vi "Register for Triggered Log State Change Event.vi"(8 "error in (no error)":errorcluster, 9 "User Data":variant, 10 "State Change Callback":refnum<vi>, 11 "Triggered Log in":refnum<class "Triggered Log.lvclass">) -> (0 "error out":errorcluster, 3 "Triggered Log out":refnum<class "Triggered Log.lvclass">)   [LabVIEW 2012, in "Triggered Log.lvclass"]
uses:
  Triggered Log.lvclass
  Triggered Log.lvclass/Triggered Log.ctl
  Triggered Log State Change Event Registration.ctl
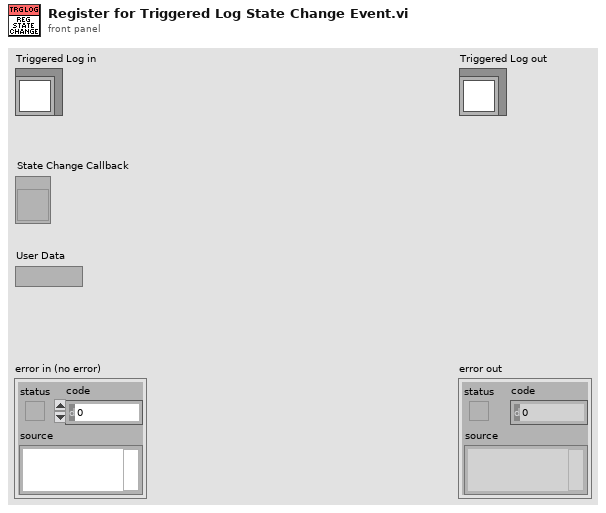
[diagram p1: front panel]
types:
  T1 = typedef "Triggered Log.lvclass/Triggered Log State Change Event Registration.ctl" = cluster{"Callback":refnum<vi>, "User Data":variant}
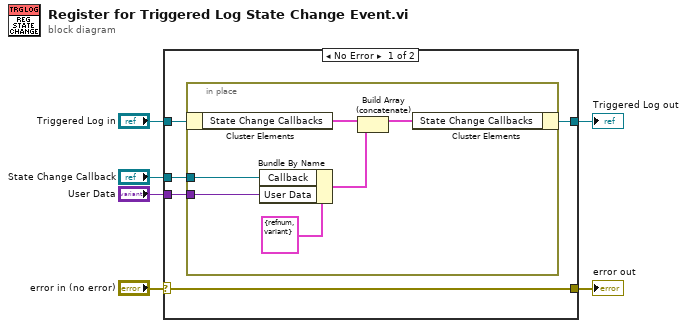
[diagram p0: block diagram]
diagram:
  n1 = case shown="No Error" "error in (no error)" {
    selector: "error in (no error)" -> [w9 w19]
    tunnel: [w9 w19] -> w5
    tunnel: [w10 w18] -> w3
    tunnel: "Triggered Log in" -> [w11 w18]
    tunnel: "State Change Callback" -> [w8 _]
    tunnel: "User Data" -> [w7 _]
    frame No Error {
      n2 = in-place {
        in-place-border: w8 -> [w14]
        in-place-border: w7 -> [w13]
        n3 = in-place-cluster #1(w11) -> ("State Change Callbacks"=w17:T1[])
        n4 = Bundle By Name(cluster=T1 {"Callback"=refnum, "User Data"=variant} ("Trigger Event Registration"), "Callback"=w14, "User Data"=w13) -> (w12:T1)
        n5 = Build Array (concatenate)(w17, w12) -> (w16:T1[])
        n6 = in-place-cluster #1("State Change Callbacks"=w16) -> (w10:refnum<class "Triggered Log.lvclass">)
      }
    }
    frame Error {
    }
  }
  "error out" <- w5
  "Triggered Log out" <- w3
